vi "BT-Android_AE_sub.vi"(0 "VISA resource name":refnum<visa-resource-name>="COM13", 1 "send data":string, 4 "存盘":bool, 5 "error in (no error)":errorcluster, 6 "End Write on Termination Character?":bool, 7 "timeout (10sec)":u32=10000, 8 "VISA buffer":i32, 10 "mode":T1(ring), 11 "Receive from Instr(bytes)\n(最好70倍数)":i32=640, 13 "file path (dialog if empty)":path=path "E:/测试数据/新芯片", 14 "baud rate":u32=57600) -> (15 "timeout?":bool=TRUE, 17 "VISA bytes now":i32, 19 "error IO":errorcluster)   [LabVIEW 2023, in "BT-Android_interface.lvlib"]
uses:
  BT-Android_interface.lvlib
  <vilib>/Instr/_visa.llb/VISA Configure Serial Port (Instr).vi
  <vilib>/Utility/file.llb/Write Delimited Spreadsheet (I64).vi
panel:
  in  "Termination Character":u8=10 format="%.0x"
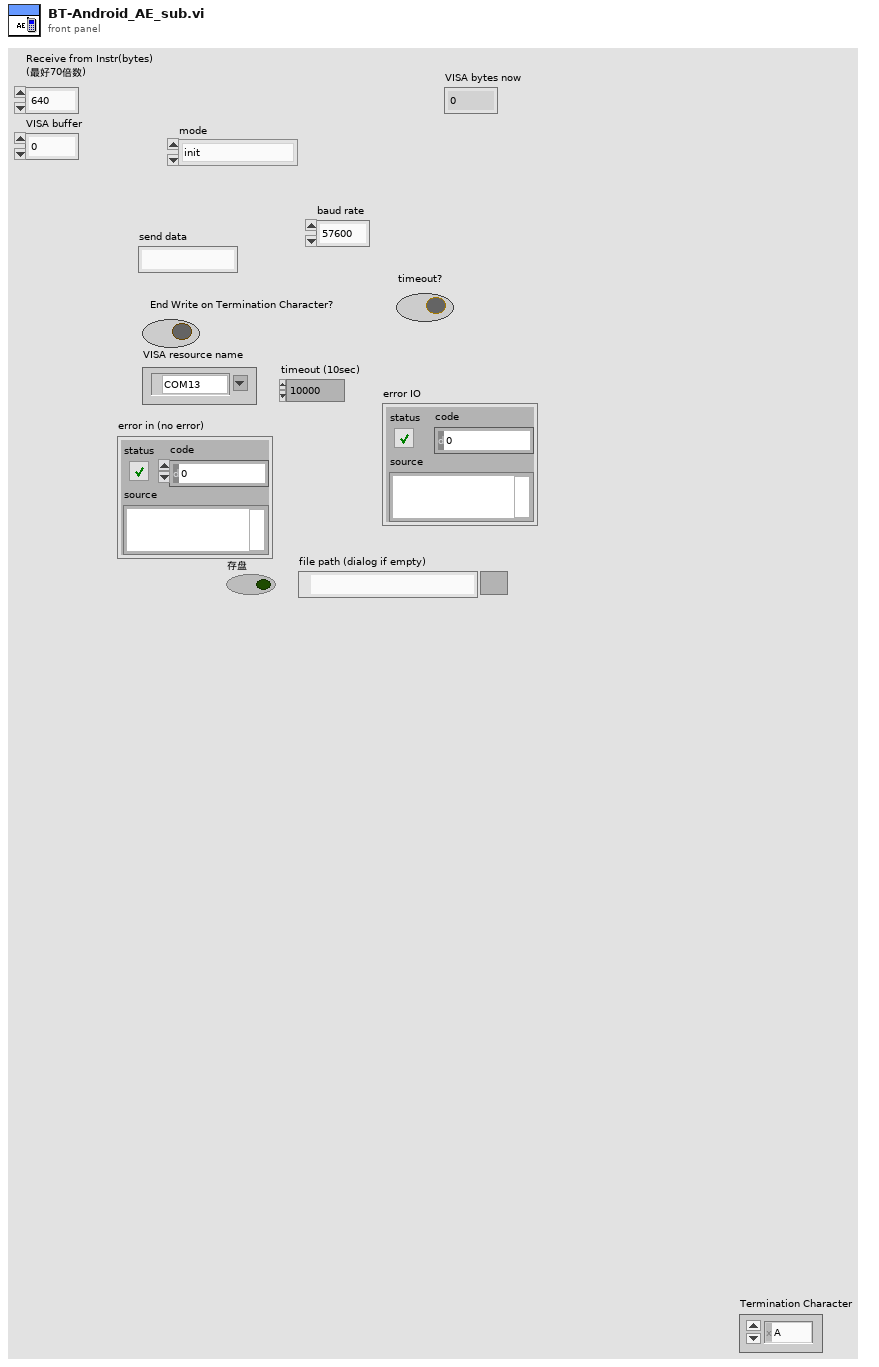
[diagram p1: front panel]
types:
  T1 = enum16{"init", "broadcast_data", "receive_data", "close", "clear_visa"}
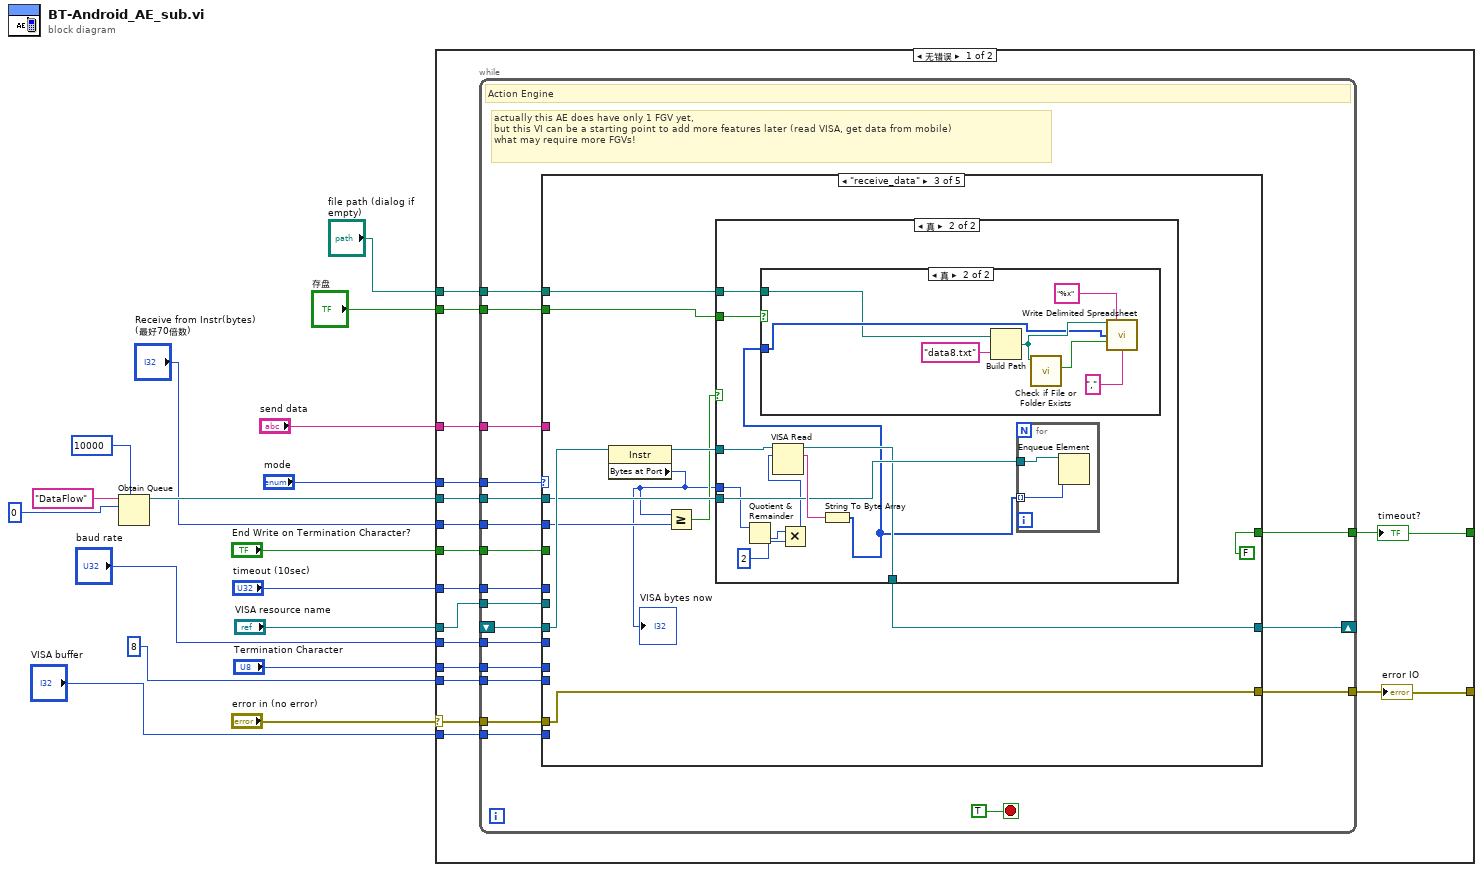
[diagram p0: block diagram]
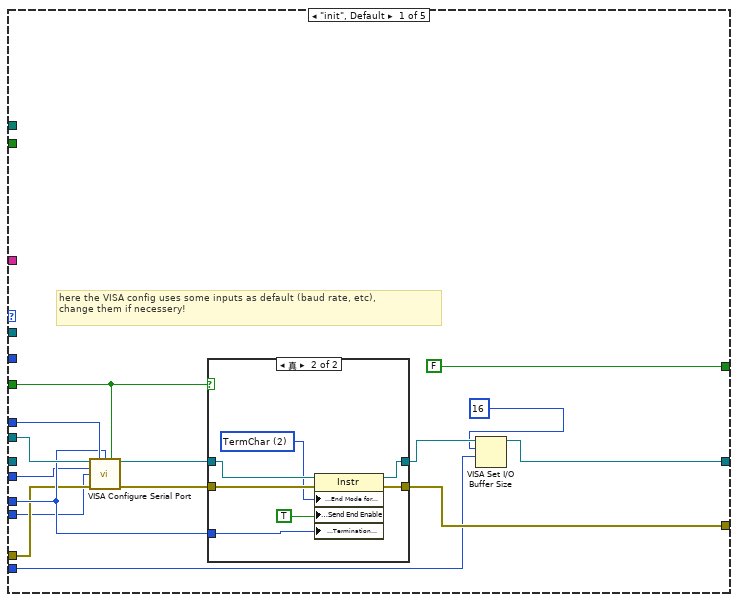
[diagram p2: hidden frame]
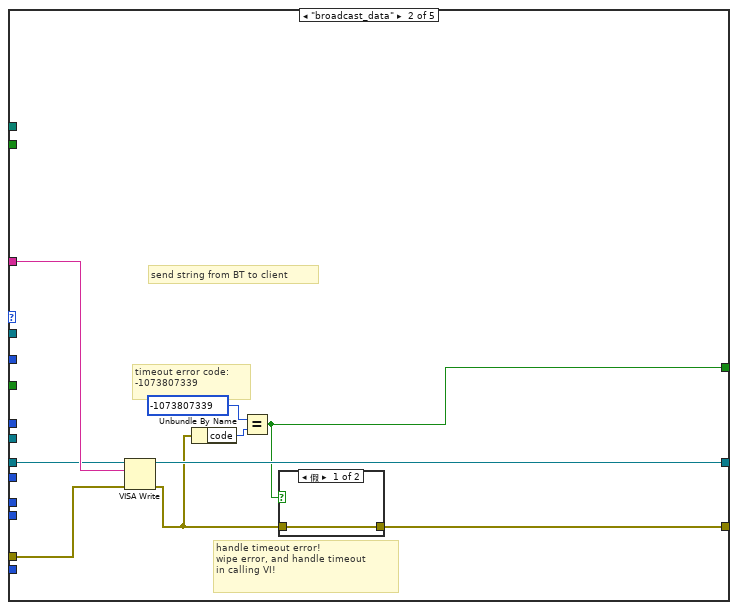
[diagram p4: hidden frame]
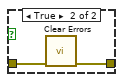
[diagram p5: hidden frame]
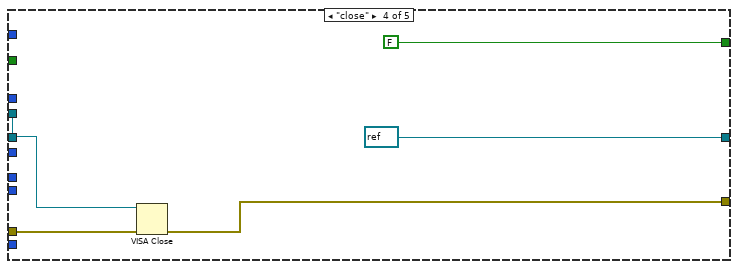
[diagram p8: hidden frame]
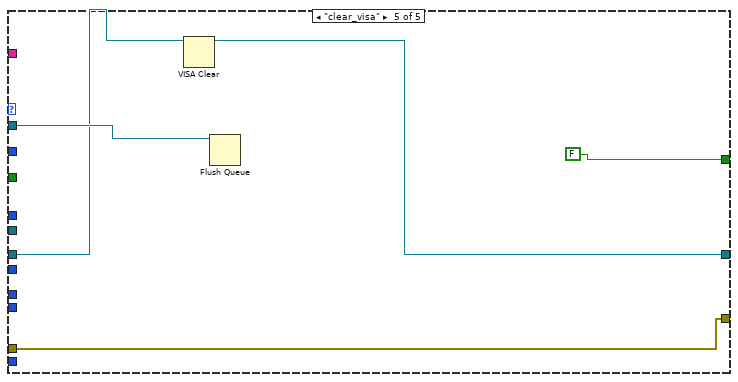
[diagram p9: hidden frame]
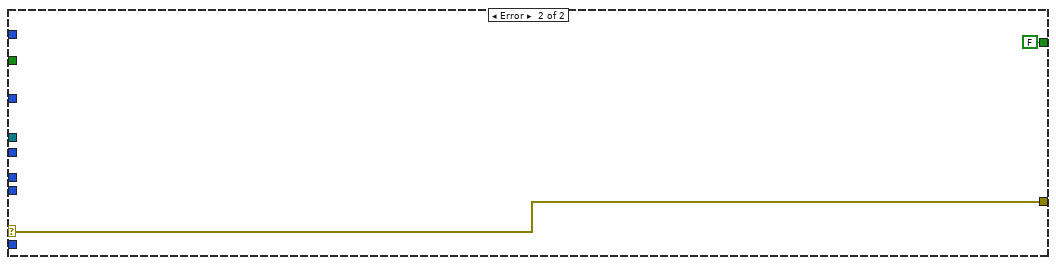
[diagram p10: hidden frame]
diagram:
  n1 = Obtain Queue(max queue size (-1, unlimited)=10000, name (unnamed)="DataFlow", element data type=u8 0) -> (queue out=w8:refnum<queue>)  [unwired: 2 in, 2 out]
  n2 = case shown="无错误" "error in (no error)" {
    selector: "error in (no error)" -> [w35 w134]
    tunnel: [w31 w134] -> w18
    tunnel: "mode" -> [w34 _]
    tunnel: "End Write on Termination Character?" -> [w33 _]
    tunnel: "timeout (10sec)" -> [w32 _]
    tunnel: "VISA resource name" -> [w27 _]
    tunnel: "Termination Character" -> [w30 _]
    tunnel: "send data" -> [w29 _]
    tunnel: [w28 FALSE] -> w11
    tunnel: w8 -> [w26 _]
    tunnel: "baud rate" -> [w25 _]
    tunnel: 8 -> [w24 _]
    tunnel: "存盘" -> [w23 _]
    tunnel: "file path (dialog if empty)" -> [w22 _]
    tunnel: "Receive from Instr(bytes)\n(最好70倍数)" -> [w21 _]
    tunnel: "VISA buffer" -> [w20 _]
    frame No Error {
      n3 = while {
        tunnel: w35 -> [w53]
        tunnel: w34 -> [w52]
        tunnel: w33 -> [w51]
        tunnel: w32 -> [w50]
        shift-right: [w49] -> _
        shift-left: _ -> [w43]
        tunnel: [w48] -> w31
        tunnel: w30 -> [w47]
        tunnel: w29 -> [w46]
        tunnel: [w45] -> w28
        tunnel: w27 -> [w44]
        tunnel: w26 -> [w42]
        tunnel: w25 -> [w41]
        tunnel: w24 -> [w40]
        tunnel: w23 -> [w39]
        tunnel: w22 -> [w38]
        tunnel: w21 -> [w37]
        tunnel: w20 -> [w36]
        stop <- TRUE stop-if-true
        # "actually this AE does have only 1 FGV yet, \nbut this VI can be a starting point to add more features later (read VISA, get data from mobile)\nwhat may require more FGVs!"
        # "Action Engine"
        n4 = case shown="\"receive_data\"" w52 {
          tunnel: w53 -> [w63 w87 w96 w127 w128]
          tunnel: w51 -> [w61 _ _ _ _]
          tunnel: w50 -> [w67 _ _ _ _]
          tunnel: w44 -> [w66 _ _ w125 _]
          tunnel: [w57 w86 w97 refnum<visa-resource-name> refnum ("VISA resource name out") w129] -> w49
          tunnel: [w65 w84 w96 w126 w128] -> w48
          tunnel: w47 -> [w64 _ _ _ _]
          tunnel: w46 -> [_ w85 _ _ _]
          tunnel: [FALSE w80 FALSE FALSE FALSE] -> w45
          tunnel: w43 -> [_ w79 w101 _ w131]
          tunnel: w42 -> [_ _ w99 _ w132]
          tunnel: w41 -> [w60 _ _ _ _]
          tunnel: w40 -> [w59 _ _ _ _]
          tunnel: w39 -> [_ _ w95 _ _]
          tunnel: w38 -> [_ _ w94 _ _]
          tunnel: w37 -> [_ _ w92 _ _]
          tunnel: w36 -> [w55 _ _ _ _]
          frame "init", Default {
            # "here the VISA config uses some inputs as default (baud rate, etc),\nchange them if necessery!"
            n5 = call-poly "VISA Configure Serial Port"("VISA resource name"=w66, "timeout (10sec)"=w67, "termination char\n(0xA = '\\n' = LF)"=w64, "Enable Termination\nChar (T)"=w61, "baud rate (9600)"=w60, "data bits (8)"=w59, "error in (no error)"=w63) -> ("VISA resource name out"=w68:refnum<visa-resource-name>, "error out"=w69:errorcluster)  [unwired: 3 in, 4 out]
            n6 = case shown="真" w61 {
              tunnel: w68 -> [w70 w78]
              tunnel: w69 -> [w71 w77]
              tunnel: [w70 w76] -> w58
              tunnel: [w71 w75] -> w65
              tunnel: w64 -> [_ w73]
              frame False {
              }
              frame True {
                w74 = u16 2 items=["None", "LastBit", "TermChar", "Break"] ("Serial Settings:Serial End Mode for Writes")
                n7 = property class="Instr"(reference=w78, error in=w77, "Serial Settings:End Mode for Writes"=w74, "Message Based Settings:Send End Enable"=TRUE, "Message Based Settings:Termination Character"=w73) -> (reference out=w76:refnum<visa-resource-name>, error out=w75:errorcluster)
              }
            }
            n8 = VISA Set I/O Buffer Size(VISA resource name=w58, mask (16)=16, size (4096)=w55) -> (VISA resource name out=w57:refnum<visa-resource-name>)  [unwired: 1 in, 1 out]
          }
          frame "broadcast_data" {
            # "send string from BT to client"
            # "handle timeout error!\nwipe error, and handle timeout\nin calling VI!"
            # "timeout error code:\n-1073807339"
            n9 = VISA Write(VISA resource name=w79, write buffer=w85, error in (no error)=w87) -> (VISA resource name out=w86:refnum<visa-resource-name>, error out=w83:errorcluster)  [unwired: 1 out]
            n10 = Unbundle By Name(w83) -> ("code"=w82:i32)
            n11 = Equal?(x=-1073807339 ("code"), y=w82) -> (x = y?=w80:bool)
            n12 = case shown="假" w80 {
              tunnel: w83 -> [w88 w90]
              tunnel: [w88 w89] -> w84
              frame False {
              }
              frame True {
                n13 = call <vilib>:"Clear Errors.vi"("error in (no error)"=w90) -> ("error out"=w89:errorcluster)  [unwired: 5 in, 1 out]
              }
            }
          }
          frame "receive_data" {
            n14 = property class="Instr"(reference=w101) -> (reference out=w100:refnum<visa-resource-name>, "Bytes at Port"=w91:u32)  [unwired: 1 in, 1 out]
            "VISA bytes now" <- w91
            n15 = Greater Or Equal?(x=w91, y=w92) -> (x >= y?=w93:bool)
            n16 = case shown="真" w93 {
              tunnel: w100 -> [w102 w113]
              tunnel: w99 -> [_ w111]
              tunnel: [w102 w110] -> w97
              tunnel: w95 -> [_ w109]
              tunnel: w94 -> [_ w108]
              tunnel: w91 -> [_ w107]
              frame False {
              }
              frame True {
                w105 = u8 2
                n17 = Quotient & Remainder(x=w107, y=w105) -> (floor(x/y)=w106:u32)  [unwired: 1 out]
                n18 = Multiply(x=w106, y=w105) -> (x*y=w104:u32)
                n19 = VISA Read(VISA resource name=w113, byte count=w104) -> (VISA resource name out=w110:refnum<visa-resource-name>, read buffer=w112:string)  [unwired: 1 in, 2 out]
                n20 = String To Byte Array(string=w112) -> (unsigned byte array=w103:u8[])
                n21 = case shown="真" w109 {
                  tunnel: w103 -> [_ w117]
                  tunnel: w108 -> [_ w116]
                  frame False {
                  }
                  frame True {
                    n22 = Build Path(base path=w116, name or relative path="data8.txt") -> (appended path=w118:path)
                    n23 = call <vilib>:"Check if File or Folder Exists.vi"("path"=w118) -> ("file or folder exists?"=w120:bool)  [unwired: 8 in, 2 out]
                    n24 = call-poly <vilib>:"Write Delimited Spreadsheet.vi"("file path (dialog if empty)"=w118, "format (%d)"="%x", "1D data"=w117, "append to file? (new file:F)"=w120, "delimiter (\\t)"=",") -> ()  [unwired: 9 in, 2 out]
                  }
                }
                n25 = for {
                  tunnel: w103 -> [w122] mode=indexing
                  tunnel: w111 -> [w121]
                  n26 = Enqueue Element(queue=w121, element=w122) -> ()  [unwired: 2 in, 3 out]
                }
              }
            }
          }
          frame "close" {
            n27 = VISA Close(VISA resource name=w125, error in (no error)=w127) -> (error out=w126:errorcluster)
          }
          frame "clear_visa" {
            n28 = VISA Clear(VISA resource name=w131) -> (VISA resource name out=w129:refnum<visa-resource-name>)  [unwired: 1 in, 1 out]
            n29 = Flush Queue(queue=w132) -> ()  [unwired: 1 in, 3 out]
          }
        }
      }
    }
    frame Error {
    }
  }
  "error IO" <- w18
  "timeout?" <- w11
